vi "mnms.vi"(0 "ROI Descriptor (Color Location 1)":T1={"Global Rectangle"=[260, 542, 2918, 2381], "Contours"=[{"ID"=enum."External", "Type"=12, "Coordinates"=[260, 542, 2918, 2381, 0]}]} {"Contours"."Type" items=["No Selection", "Point", "Line", "Rectangle", "Oval", "Polygon", "Freehand Region", "Annulus", "Unused2", "Unused3", "Broken Line", "Freehand Line", "Rotated Rectangle"]}, 1 "Number of Matches Requested (Color Location 1)":i32=12, 2 "Minimum Match Score (Color Location 1)":sgl=700.0, 7 "error in":errorcluster) -> (20 "Matches (Color Location 1)":T3(array[cluster]) {"Bounding Box"."y" format="%.2f"; "Bounding Box"."x" format="%.2f"; "Position"."y" format="%.2f"; "Position"."x" format="%.2f"; "Score" format="%.2f"; "Scale" format="%.2f"; "Angle" format="%.2f"}, 21 "Number of Matches (Color Location 1)":i32, 27 "error out":errorcluster)   [LabVIEW 2017]
uses:
  <vilib>/vision/NI_Vision_Development_Module.lvlib
panel:
  out "Image Out":T2(plugin-control)
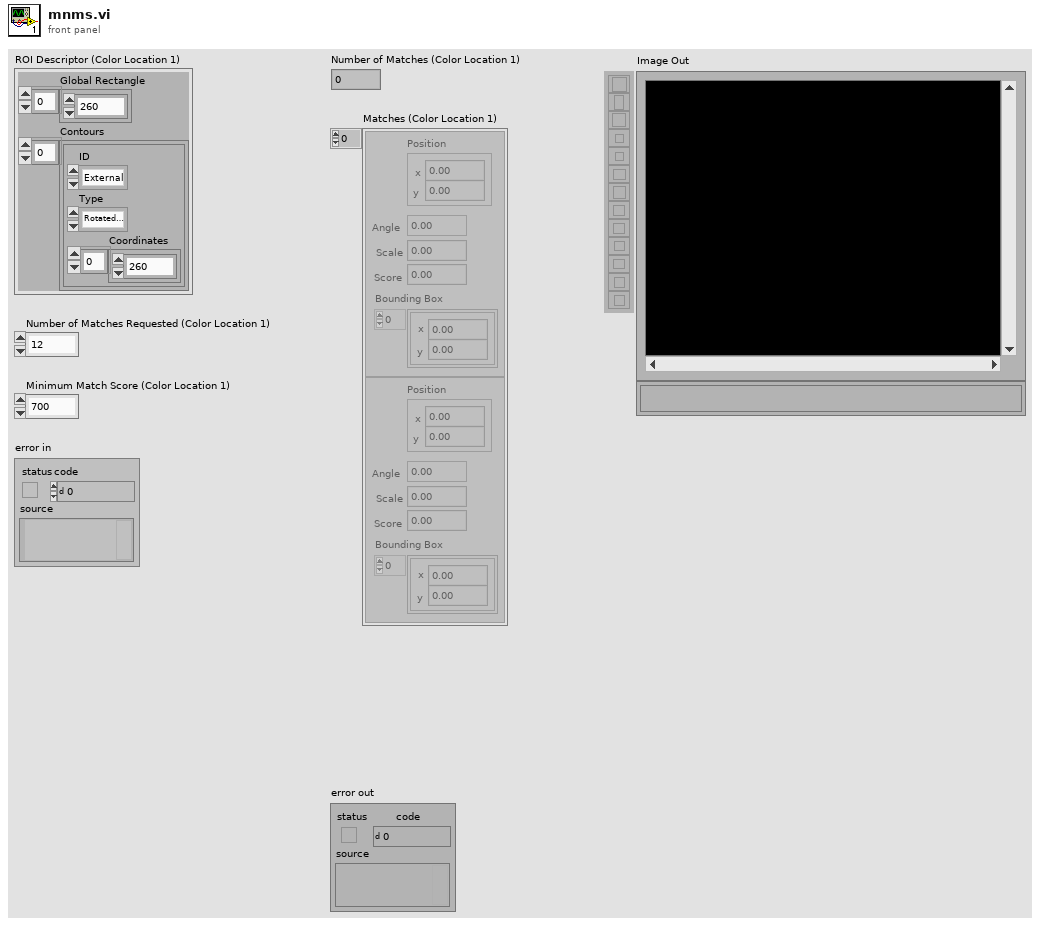
[diagram p1: front panel]
types:
  T1 = cluster{"Global Rectangle":i32[], "Contours":cluster{"ID":enum32{"External", "Internal"}, "Type":u32, "Coordinates":i32[]}[]}
  T2 = typedef "IMAQ Image.ctl" = refnum<image>
  T3 = cluster{"Position":cluster{"x":sgl, "y":sgl}, "Angle":sgl, "Scale":sgl, "Score":sgl, "Bounding Box":cluster{"x":sgl, "y":sgl}[]}[]
  T4 = typedef "Image Type" = u32
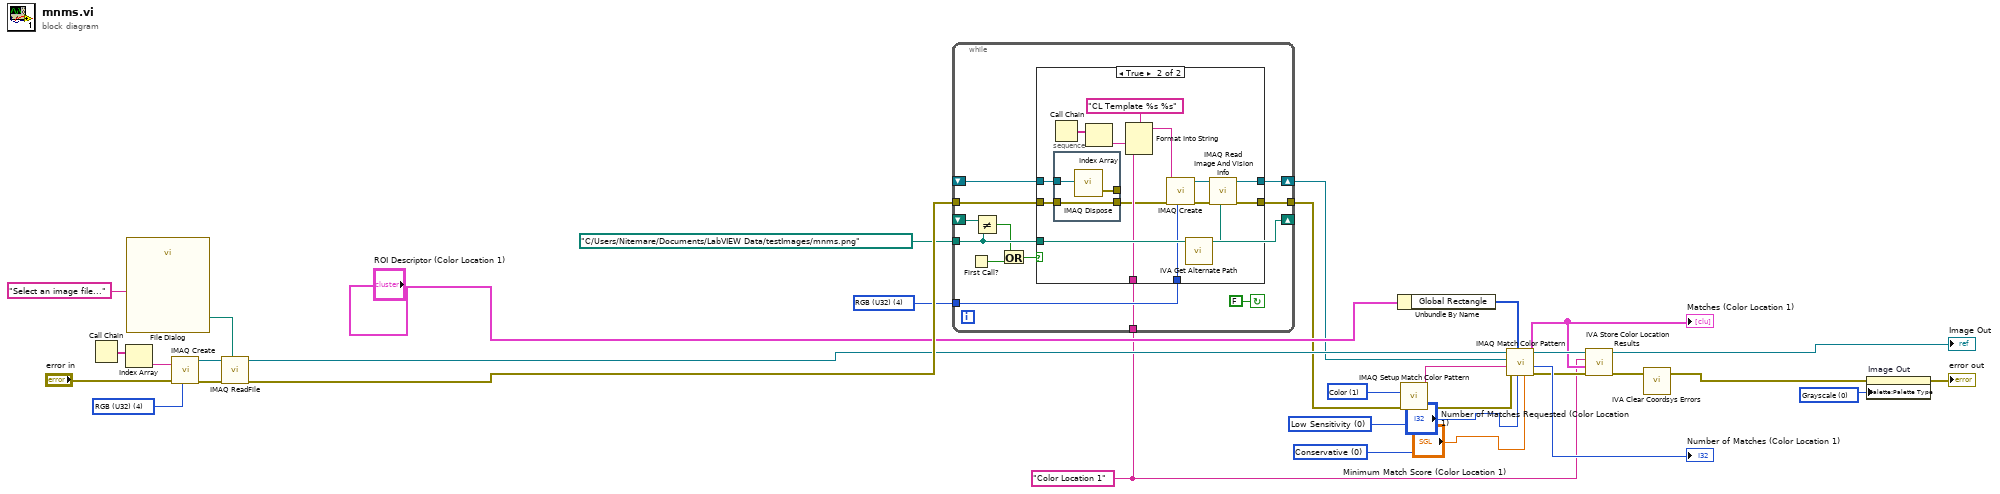
[diagram p0: block diagram]
diagram:
  w1 = u32 0 items=["Grayscale", "Binary", "Gradient", "Rainbow", "Temperature", "User Defined", "Binary 16 Bit", "Gradient 16 Bit", "Rainbow 16 Bit", "Temperature 16 Bit", "User Defined 16 Bit"] ("Palette Type")
  w11 = "Color Location 1" ("Step Name")
  w16 = T4 4 items=["Grayscale (U8)", "Grayscale (I16)", "Grayscale (SGL)", "Complex (CSG)", "RGB (U32)", "HSL (U32)", "RGB (U64)"] ("Image Type")
  w18 = u32 0 items=["Conservative", "Balance", "Aggressive", "Very Aggressive"] ("Search Strategy")
  w19 = u32 0 items=["Low Sensitivity", "Medium Sensitivity", "High Sensitivity"] ("Color Sensitivity")
  w20 = u32 1 items=["Color and Shape", "Color", "Shape"] ("Match Feature Mode")
  w24 = T4 4 items=["Grayscale (U8)", "Grayscale (I16)", "Grayscale (SGL)", "Complex (CSG)", "RGB (U32)", "HSL (U32)", "RGB (U64)", "Grayscale (U16)"] ("Image Type")
  n1 = Call Chain() -> (call chain=w28:string[])
  n2 = Index Array(array=w28) -> (element=w27:string)  [unwired: 1 in]
  n3 = call "File Dialog"("prompt"="Select an image file...") -> ("selected path"=w25:path)  [unwired: 6 in, 8 out]
  n4 = call "IMAQ Create"("Image Name"=w27, "Image Type"=w24, "error in (no error)"="error in") -> ("New Image"=w31:T2, "error out"=w30:errorcluster)  [unwired: 1 in, 1 out]
  n5 = call "IMAQ ReadFile"("File Path"=w25, "error in (no error)"=w30, "Image"=w31) -> ("error out"=w32:errorcluster, "Image Out"=w13:T2)  [unwired: 2 in, 5 out]
  n6 = while {
    shift-right: [w44] -> w7
    shift-left: _ -> [w43]
    tunnel: [w41] -> w6
    tunnel: w32 -> [w40]
    tunnel: path "C:/Users/Nitemare/Documents/LabVIEW Data/testImages/mnms.png" ("File Path") -> [w36]
    tunnel: w16 -> [w39]
    tunnel: w11 -> [w38]
    shift-right: [w36] -> _
    shift-left: _ -> [w37]
    stop <- FALSE continue-if-true
    n7 = First Call?() -> (First Call?: T/F=w35:bool)
    n8 = Not Equal?(x=w37, y=w36) -> (x != y?=w34:bool)
    n9 = Or(x=w34, y=w35) -> (x .or. y?=w33:bool)
    n10 = case shown="True" w33 {
      tunnel: [w46 w59] -> w44
      tunnel: w43 -> [w46 w51]
      tunnel: [w45 w56] -> w41
      tunnel: w40 -> [w45 w50]
      tunnel: w39 -> [_ w55]
      tunnel: w38 -> [_ w52]
      tunnel: w36 -> [_ w48]
      frame False {
      }
      frame True {
        n11 = Call Chain() -> (call chain=w54:string[])
        n12 = stacked-sequence {
          tunnel: w51 -> [w64]
          tunnel: w50 -> [w63]
          tunnel: [w63] -> w49
          tunnel: [w62] -> _
          frame #0 {
            n13 = call "IMAQ Dispose"("Image"=w64) -> ("error out"=w62:errorcluster)  [unwired: 2 in, 3 out]
          }
        }
        n14 = Index Array(array=w54) -> (element=w53:string)  [unwired: 1 in]
        n15 = Format Into String(format string="CL Template %s %s" ("Image Name"), w53, w52) -> (resulting string=w61:string)  [unwired: 2 in, 1 out]
        n16 = call "IMAQ Create"("Image Name"=w61, "Image Type"=w55, "error in (no error)"=w49) -> ("New Image"=w58:T2, "error out"=w57:errorcluster)  [unwired: 1 in, 1 out]
        n17 = call <vilib>:"IVA Get Alternate Path.vi"("Path In"=w48) -> ("Path Out"=w47:path)  [unwired: 10 out]
        n18 = call "IMAQ Read Image And Vision Info"("File Path"=w47, "error in (no error)"=w57, "Image"=w58) -> ("error out"=w56:errorcluster, "Image Out"=w59:T2)  [unwired: 1 in, 6 out]
      }
    }
  }
  n19 = Unbundle By Name("ROI Descriptor (Color Location 1)") -> ("Global Rectangle"=w8:i32[])
  n20 = call "IMAQ Setup Match Color Pattern"("Match Feature Mode"=w20, "error in (no error)"=w6, "Color Sensitivity"=w19, "Search Strategy"=w18) -> ("Match Color Pattern Setup Data"=w10:string, "error out"=w9:errorcluster)  [unwired: 5 in, 5 out]
  n21 = call "IMAQ Match Color Pattern"("Minimum Match Score"="Minimum Match Score (Color Location 1)", "Number of Matches Requested"="Number of Matches Requested (Color Location 1)", "Optional Rectangle"=w8, "error in (no error)"=w9, "Match Color Pattern Setup Data"=w10, "Template Image"=w7, "Image"=w13) -> ("error out"=w14:errorcluster, "Number of Matches"=→"Number of Matches (Color Location 1)":i32, "Matches"=w12:T3)  [unwired: 2 out]
  "Matches (Color Location 1)" <- w12
  n22 = call <vilib>:"IVA Store Color Location Results.vi"("error in (no error)"=w14, "Matches"=w12, "Step Name"=w11, "Image in"=w13) -> ("error out"=w5:errorcluster, "Image dup"=→"Image Out":T2)  [unwired: 6 out]
  n23 = call <vilib>:"IVA Clear Coordsys Errors.vi"("error in (no error)"=w5) -> ("error out"=w4:errorcluster)  [unwired: 10 in]
  n24 = property on="Image Out" class="ImageControl"(error in=w4, "Palette:Palette Type"=w1) -> (error out=→"error out":errorcluster)  [unwired: 1 in, 1 out]
